vi "PH_Timing.panel.vi"(0 "object ref":refnum<vi>, 5 "error in (no error)":errorcluster) -> (19 "error out":errorcluster)   [LabVIEW 2014, in "PH_Timing.lvlib"]
doc: "This a GUI.\n\nLicense Agreement for this software:\n\nCopyright (C)\nGesellschaft für Schwerionenforschung, GSI\nPlanckstr. 1\n64291 Darmstadt\nGermany\n\nContact: D.Beck@gsi.de \n\nThis program is free software; you can redistribute it and/or modify it under the terms of the GNU General Public License as published by the Free Software Foundation; either version 2 of the license, or (at your option) any later version.\n\nThis program is distributed in the hope that it will be useful, but WITHOUT ANYW ARRANTY; without even the implied warranty of MERCHANTABILITY or FITNESS FOR A PARTICULAR PURPOSE. See the GNU General License for more details (http://www.gnu.org).\n\nGesellschaft für Schwerionenforschung, GSI\nPlanckstr. 1, 64291 Darmstadt, Germany\nFor all questions and ideas contact: M.Richter@gsi.de, H.Brand@gsi.de or D.Beck@gsi.de.\nLast update: 18-DEC-2002"
uses:
  PH_Timing.lvlib
  PH_StatusHandler/PH_StatusHandler.GUI element.ctl
  PH_Timing.PU Info.ctl
  PH_Timing.GateGen.ctl
  PH_Timing.Roughtuner.ctl
  PH_Timing.0.5HzGater.ctl
  PH_Timing.Slow Trigger Settings.ctl
  PH_Timing.Timing Mode.ctl
  PH_Timing.ns Generator.ctl
  instr.lib/Stanford Research DG645/Driver/Channel.ctl
  PH_SRDG645/PH_SRDG645.Channel Settings.ctl
  PH_Timing.Phase FEs.ctl
  CSCore/CSObj/CSObj.lvlib
  PH_Common/PH_Common.lvlib
  PH_Class/PH_Class.lvlib
  PH_StatusHandler/PH_StatusHandler.lvlib
  instr.lib/Stanford Research DG645/Stanford Research DG645 - Driver.lvlib
  PH_SRDG645/PH_SRDG645.lvlib
panel:
  out "FE Phase":T1 {"Phase" format="%#_12p"}
  out "Timing_ns_Ring_Regen_GD":u32(colorbox)=6618880 caption="ns Ring Regen"
  out "Timing Mode":T2 {"T2" min=0 max=6000 step=2}
  out "Slow Trigger Settings":T3
  out "Timing_0-5HzGater_GD":u32(colorbox)=6618880 caption="0.5Hz Gater"
  out "Timing_Roughtuner_GD":u32(colorbox)=6618880 caption="Roughtuner"
  out "Interlock Bypass":u32(colorbox)=6618880
  in  "Tab Control":T4(tab)
  out "ns Generator Settings":T5={"Instance"="N/A", "Phase fs / ns FE"={"Channel"=0, "Settings"={"Delay [s]"=0.0, "relative to"=0}}} {"Phase fs / ns FE"."Settings"."relative to" items=["T0", "T1", "A", "B", "C", "D", "E", "F", "G", "H"]; "Phase fs / ns FE"."Settings"."Delay [s]" format="%#_12p"; "Phase fs / ns FE"."Channel" items=["T0", "T1", "A", "B", "C", "D", "E", "F", "G", "H"]}
  out "Roughtuner Settings":T8={"Instance"="N/A", "Phase PHELIX / UNILAC"={"Channel"=0, "relative to"=0, "Delay [ms]"=0.0}, "Pulse Length"={"Channel"=0, "relative to"=0, "Delay [ms]"=0.0}, "Trigger"={"externally?"=FALSE, "Rate [Hz]"=0.0}} {"Pulse Length"."Delay [ms]" format="%#_8g"; "Pulse Length"."relative to" items=["T0", "A", "B", "AB", "C", "D", "CD"]; "Pulse Length"."Channel" items=["T0", "A", "B", "AB", "C", "D", "CD"]; "Phase PHELIX / UNILAC"."Delay [ms]" format="%#_8g"; "Phase PHELIX / UNILAC"."relative to" items=["T0", "A", "B", "AB", "C", "D", "CD"]; "Phase PHELIX / UNILAC"."Channel" items=["T0", "A", "B", "AB", "C", "D", "CD"]}
  out "Info 0,5Hz Gater":T9={"Instance"="N/A", "Channel ns FE Delay"=1, "Channel 0.5Hz"=1, "Width ns FE Delay"=1.0, "Width 0.5Hz"=1.0, "Delay ns FE Delay"=0.0, "Delay 0.5Hz"=0.0, "ns FE Delay active"=FALSE, "0.5Hz activ"=FALSE, "ns FE Delay inverted"=FALSE, "0.5Hz inverted"=FALSE} {"Channel ns FE Delay" items=["System (To)", "Channel A", "Channel B", "Channel C", "Channel D", "Channel E", "Channel F", "Channel G", "Channel H"]; "Channel 0.5Hz" items=["System (To)", "Channel A", "Channel B", "Channel C", "Channel D", "Channel E", "Channel F", "Channel G", "Channel H"]}
  out "Info Gate Generator":T10={"Instance"="N/A", "Channel Gate"=1, "Channel T2"=1, "Width Gate"=1.0, "Width T2"=1.0, "Delay Gate"=0.0, "Delay T2"=0.0, "Gate activ"=FALSE, "T2 activ"=FALSE, "System Mode"=enum."Normal"} {"Channel Gate" items=["System (To)", "Channel A", "Channel B", "Channel C", "Channel D", "Channel E", "Channel F", "Channel G", "Channel H"]; "Channel T2" items=["System (To)", "Channel A", "Channel B", "Channel C", "Channel D", "Channel E", "Channel F", "Channel G", "Channel H"]}
  out "PU PA 45-DP":T11={"Act CH?"=FALSE, "GD"="N/A", "CH"=1, "Delay"=99999.0, "active"=FALSE, "in Use?"=FALSE} {"CH" items=["System (To)", "Channel A", "Channel B", "Channel C", "Channel D", "Channel E", "Channel F", "Channel G", "Channel H"]; "Delay" format="%#_7f"}
  out "PU PA 45-MAIN":T11={"Act CH?"=FALSE, "GD"="N/A", "CH"=1, "Delay"=99999.0, "active"=FALSE, "in Use?"=FALSE} {"CH" items=["System (To)", "Channel A", "Channel B", "Channel C", "Channel D", "Channel E", "Channel F", "Channel G", "Channel H"]; "Delay" format="%#_7f"}
  out "PU PA 45-PILC":T11={"Act CH?"=FALSE, "GD"="N/A", "CH"=1, "Delay"=99999.0, "active"=FALSE, "in Use?"=FALSE} {"CH" items=["System (To)", "Channel A", "Channel B", "Channel C", "Channel D", "Channel E", "Channel F", "Channel G", "Channel H"]; "Delay" format="%#_7f"}
  out "PU PA 19-2":T11={"Act CH?"=FALSE, "GD"="N/A", "CH"=1, "Delay"=99999.0, "active"=FALSE, "in Use?"=FALSE} {"CH" items=["System (To)", "Channel A", "Channel B", "Channel C", "Channel D", "Channel E", "Channel F", "Channel G", "Channel H"]; "Delay" format="%#_7f"}
  out "PU PA 19-1":T11={"Act CH?"=FALSE, "GD"="N/A", "CH"=1, "Delay"=99999.0, "active"=FALSE, "in Use?"=FALSE} {"CH" items=["System (To)", "Channel A", "Channel B", "Channel C", "Channel D", "Channel E", "Channel F", "Channel G", "Channel H"]; "Delay" format="%#_7f"}
  out "PU MA 5":T11={"Act CH?"=FALSE, "GD"="N/A", "CH"=1, "Delay"=99999.0, "active"=FALSE, "in Use?"=FALSE} {"CH" items=["System (To)", "Channel A", "Channel B", "Channel C", "Channel D", "Channel E", "Channel F", "Channel G", "Channel H"]; "Delay" format="%#_7f"}
  out "PU MA 4":T11={"Act CH?"=FALSE, "GD"="N/A", "CH"=1, "Delay"=99999.0, "active"=FALSE, "in Use?"=FALSE} {"CH" items=["System (To)", "Channel A", "Channel B", "Channel C", "Channel D", "Channel E", "Channel F", "Channel G", "Channel H"]; "Delay" format="%#_7f"}
  out "PU MA 3":T11={"Act CH?"=FALSE, "GD"="N/A", "CH"=1, "Delay"=99999.0, "active"=FALSE, "in Use?"=FALSE} {"CH" items=["System (To)", "Channel A", "Channel B", "Channel C", "Channel D", "Channel E", "Channel F", "Channel G", "Channel H"]; "Delay" format="%#_7f"}
  out "PU MA 2":T11={"Act CH?"=FALSE, "GD"="N/A", "CH"=1, "Delay"=99999.0, "active"=FALSE, "in Use?"=FALSE} {"CH" items=["System (To)", "Channel A", "Channel B", "Channel C", "Channel D", "Channel E", "Channel F", "Channel G", "Channel H"]; "Delay" format="%#_7f"}
  out "PU MA 1":T11={"Act CH?"=FALSE, "GD"="N/A", "CH"=1, "Delay"=99999.0, "active"=FALSE, "in Use?"=FALSE} {"CH" items=["System (To)", "Channel A", "Channel B", "Channel C", "Channel D", "Channel E", "Channel F", "Channel G", "Channel H"]; "Delay" format="%#_7f"}
  out "PA MA FR":T11={"Act CH?"=FALSE, "GD"="N/A", "CH"=1, "Delay"=99999.0, "active"=FALSE, "in Use?"=FALSE} {"CH" items=["System (To)", "Channel A", "Channel B", "Channel C", "Channel D", "Channel E", "Channel F", "Channel G", "Channel H"]; "Delay" format="%#_7f"}
  out "State Sequencer":string caption="State PU"
  out "Timing_PP_2_GD":u32(colorbox)=6618880 caption="PP 2"
  out "Timing_PP_1_GD":u32(colorbox)=6618880 caption="PP 1"
  out "Status":T12 caption="Enabling State"
  in  "Delete":bool
  out "Timing_GateGen_GD":u32(colorbox)=6618880 caption="GateGen"
  in  "Exit":bool
  # "PCS"
  # "3.40"
  # "AND ns FE Delay"
  # "AND 0.5 Hz"
  # "Gate"
  # "T2"
  # "s"
  # "s"
  # "s"
  # "s"
  # "s"
  # "s"
  # "s"
  # "s"
  # "s"
  # "s"
  # "s"
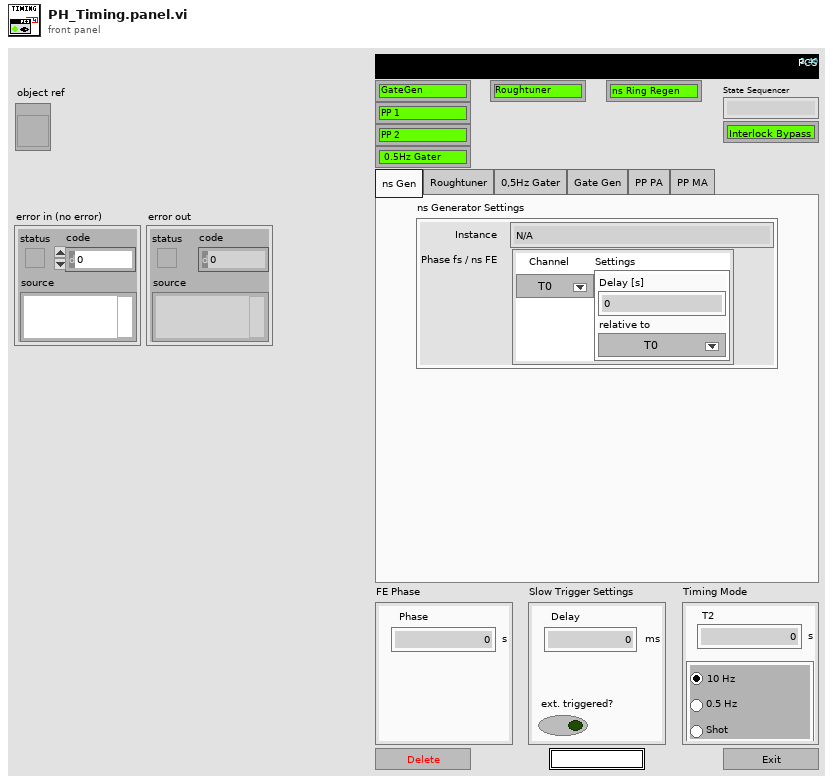
[diagram p1: front panel]
types:
  T1 = typedef "PH_Timing.lvlib/PH_Timing.Phase FEs.ctl" = cluster{"Phase":dbl}
  T2 = typedef "PH_Timing.lvlib/PH_Timing.Timing Mode.ctl" = cluster{"T2":i16, "Modeselector":enum32{"10 Hz", "0.5 Hz", "Shot"}}
  T3 = typedef "PH_Timing.lvlib/PH_Timing.Slow Trigger Settings.ctl" = cluster{"Delay":dbl, "externally triggered?":bool}
  T4 = enum32{"ns Gen", "Roughtuner", "0,5Hz Gater", "Gate Gen", "PP PA", "PP MA"}
  T5 = typedef "PH_Timing.lvlib/PH_Timing.ns Generator.ctl" = cluster{"Instance":string, "Phase fs / ns FE":cluster{"Channel":T6, "Settings":T7}}
  T6 = typedef "Stanford Research DG645 - Driver.lvlib/Channel.ctl" = i32
  T7 = typedef "PH_SRDG645.lvlib/PH_SRDG645.Channel Settings.ctl" = cluster{"Delay [s]":dbl, "relative to":i32}
  T8 = typedef "PH_Timing.lvlib/PH_Timing.Roughtuner.ctl" = cluster{"Instance":string, "Phase PHELIX / UNILAC":cluster{"Channel":u16, "relative to":u16, "Delay [ms]":dbl}, "Pulse Length":cluster{"Channel":u16, "relative to":u16, "Delay [ms]":dbl}, "Trigger":cluster{"externally?":bool, "Rate [Hz]":dbl}}
  T9 = typedef "PH_Timing.lvlib/PH_Timing.0.5HzGater.ctl" = cluster{"Instance":string, "Channel ns FE Delay":i32, "Channel 0.5Hz":i32, "Width ns FE Delay":dbl, "Width 0.5Hz":dbl, "Delay ns FE Delay":dbl, "Delay 0.5Hz":dbl, "ns FE Delay active":bool, "0.5Hz activ":bool, "ns FE Delay inverted":bool, "0.5Hz inverted":bool}
  T10 = typedef "PH_Timing.lvlib/PH_Timing.GateGen.ctl" = cluster{"Instance":string, "Channel Gate":i32, "Channel T2":i32, "Width Gate":dbl, "Width T2":dbl, "Delay Gate":dbl, "Delay T2":dbl, "Gate activ":bool, "T2 activ":bool, "System Mode":enum16{"Normal", "Single", "Burst", "Duty Cycle"}}
  T11 = typedef "PH_Timing.lvlib/PH_Timing.PU Info.ctl" = cluster{"Act CH?":bool, "GD":string, "CH":i32, "Delay":dbl, "active":bool, "in Use?":bool}
  T12 = typedef "PH_StatusHandler.lvlib/PH_StatusHandler.GUI element.ctl" = u16
  T13 = cluster{"MA PU 1":refnum<vi>, "MA PU 2":refnum<vi>, "MA PU 3":refnum<vi>, "MA PU 4":refnum<vi>, "MA PU 5":refnum<vi>, "MA FR":refnum<vi>, "PA 19mm 1":refnum<vi>, "PA 19mm 2":refnum<vi>, "PA 45mm PILC":refnum<vi>, "PA 45mm MAIN":refnum<vi>, "PA 45mm DP":refnum<vi>}
  T14 = typedef "PH_Timing.lvlib/PH_Timing.PU Data.ctl" = cluster{"linked?":bool, "Data":T11, "GD":cluster{"Device Status":T15, "linked?":bool}, "GUI Ref":refnum<vi>, "PU":T16}
  T15 = typedef "PH_StatusHandler.lvlib/PH_StatusHandler.Status.ctl" = i16
  T16 = typedef "PH_PP_Common.lvlib/PH_PP_Common.PUs.ctl" = enum16{"no Info", "PA-19mm-1", "PA-19mm-2", "PA-45mm-PILC", "PA-45mm-MAIN", "MA-PU-1", "MA-PU-2", "MA-PU-3", "MA-PU-4", "MA-PU-5", "MA-PU-6", "MA-FR", "MA-PILC", "PA-45mm-DP"}
  T17 = typedef "PH_Timing.lvlib/PH_Timing.i attribute.ctl" = cluster{"Sequencer":cluster{"linked?":bool, "Proc State":string, "Ref State":refnum<vi>}, "Gate Generator":cluster{"GD":cluster{"Device Status":T15, "linked?":bool}, "Settings":T10, "GUI Ref":refnum<vi>}, "Interlock Bypass":cluster{"Instancename":string, "Switch linked?":bool, "Device Status":T15, "Ref Status":refnum<vi>}, "Roughtuner":cluster{"Settings":T8, "GUI Ref":refnum<vi>, "GD":cluster{"Device Status":T15, "linked?":bool}}, "0,5Hz Gater":cluster{"Settings":T9, "GUI Ref":refnum<vi>, "GD":cluster{"Device Status":T15, "linked?":bool}}, "Slow Trigger":cluster{"Settings":T3, "GUI Ref":refnum<vi>, "Service ID Delay":i32, "Service ID Ext Trig":i32, "Wanted Settings":T3}, "Timing Mode":cluster{"Mode":T2, "GUI Ref":refnum<vi>, "Service ID T2":i32, "Service ID Mode":i32, "Wanted Mode":T2}, "ns Generator":cluster{"Settings":T5, "ns Generator Settings":refnum<vi>, "GD":cluster{"Device Status":T15, "linked?":bool}}, "Phase FEs":cluster{"Settings":T1, "GUI Ref":refnum<vi>, "Service ID Phase":i32, "Wanted Settings":T1}, "GD GUI Refs":refnum<vi>[], "Heads":T14[], "GUI Ref Delete":refnum<vi>}
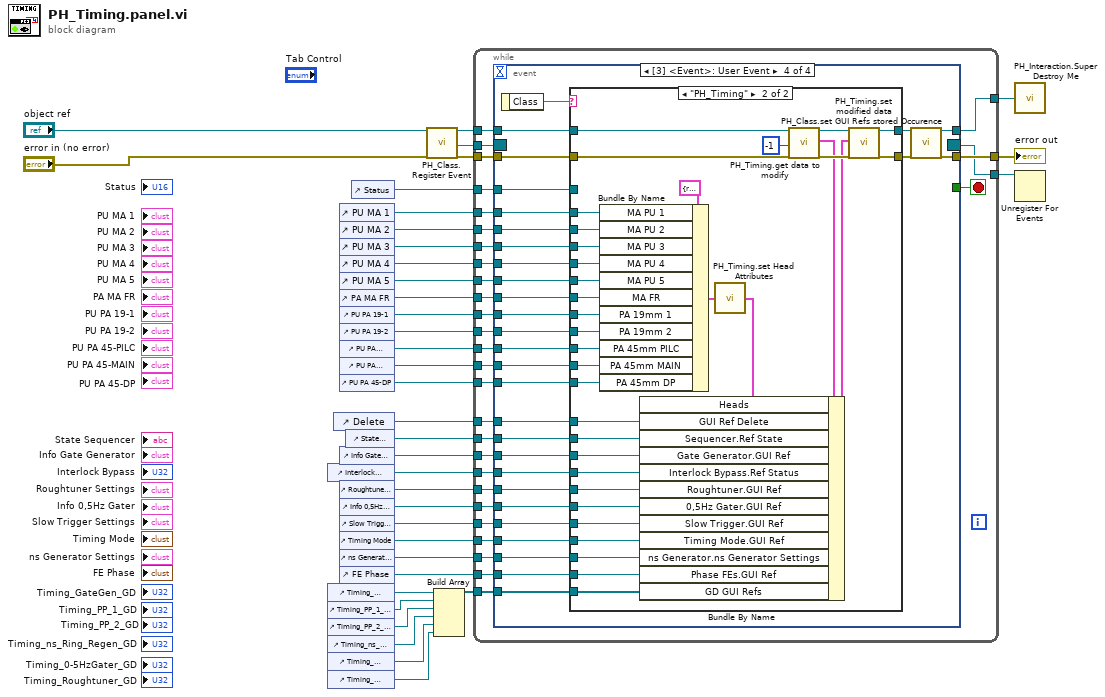
[diagram p0: block diagram]
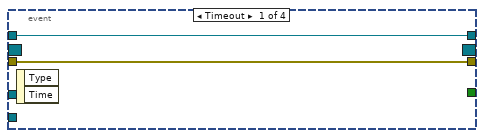
[diagram p2: hidden frame]
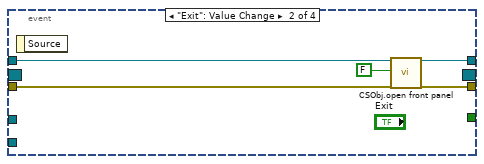
[diagram p3: hidden frame]
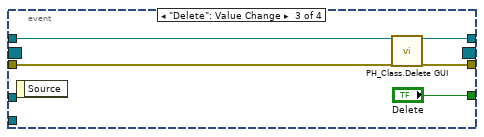
[diagram p4: hidden frame]
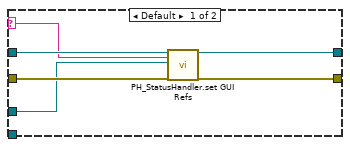
[diagram p5: hidden frame]
diagram:
  n1 = control-ref of="Interlock Bypass"() -> (w9:refnum<vi>)
  n2 = control-ref of="Timing_GateGen_GD"() -> (w37:refnum<vi>)
  n3 = control-ref of="Timing_PP_1_GD"() -> (w36:refnum<vi>)
  n4 = control-ref of="Timing_PP_2_GD"() -> (w35:refnum<vi>)
  n5 = control-ref of="Timing_ns_Ring_Regen_GD"() -> (w31:refnum<vi>)
  n6 = control-ref of="Timing_0-5HzGater_GD"() -> (w32:refnum<vi>)
  n7 = control-ref of="Timing_Roughtuner_GD"() -> (w30:refnum<vi>)
  n8 = control-ref of="Delete"() -> (w12:refnum<vi>)
  n9 = control-ref of="PU MA 1"() -> (w23:refnum<vi>)
  n10 = control-ref of="PU MA 2"() -> (w22:refnum<vi>)
  n11 = control-ref of="PU MA 3"() -> (w21:refnum<vi>)
  n12 = control-ref of="PU MA 4"() -> (w20:refnum<vi>)
  n13 = control-ref of="PU MA 5"() -> (w19:refnum<vi>)
  n14 = control-ref of="PA MA FR"() -> (w18:refnum<vi>)
  n15 = control-ref of="PU PA 19-1"() -> (w17:refnum<vi>)
  n16 = control-ref of="PU PA 19-2"() -> (w16:refnum<vi>)
  n17 = control-ref of="PU PA 45-PILC"() -> (w15:refnum<vi>)
  n18 = control-ref of="PU PA 45-MAIN"() -> (w14:refnum<vi>)
  n19 = control-ref of="PU PA 45-DP"() -> (w13:refnum<vi>)
  n20 = control-ref of="Info Gate Generator"() -> (w10:refnum<vi>)
  n21 = control-ref of="Roughtuner Settings"() -> (w8:refnum<vi>)
  n22 = control-ref of="Info 0,5Hz Gater"() -> (w7:refnum<vi>)
  n23 = control-ref of="Slow Trigger Settings"() -> (w6:refnum<vi>)
  n24 = control-ref of="Timing Mode"() -> (w5:refnum<vi>)
  n25 = control-ref of="ns Generator Settings"() -> (w4:refnum<vi>)
  n26 = control-ref of="FE Phase"() -> (w3:refnum<vi>)
  n27 = control-ref of="State Sequencer"() -> (w11:refnum<vi>)
  n28 = control-ref of="Status"() -> (w1:refnum<vi>)
  n29 = call "PH_Class.Register Event.vi"("i ref in"="object ref", "error in (no error)"="error in (no error)") -> ("i ref out"=w29:refnum<vi>, "Event Registration Refnum"=w27:refnum<event-registration>, "error out"=w28:errorcluster)  [unwired: 15 in]
  n30 = Build Array(w37, w36, w35, w31, w32, w30) -> (w2:refnum<vi>[])
  n31 = while {
    tunnel: w29 -> [w64]
    tunnel: [w63] -> w34
    tunnel: w28 -> [w66]
    tunnel: [w65] -> w33
    tunnel: w27 -> [w62]
    tunnel: [w61] -> w26
    tunnel: w23 -> [w60]
    tunnel: w22 -> [w59]
    tunnel: w21 -> [w58]
    tunnel: w20 -> [w57]
    tunnel: w19 -> [w56]
    tunnel: w18 -> [w55]
    tunnel: w17 -> [w54]
    tunnel: w16 -> [w53]
    tunnel: w15 -> [w52]
    tunnel: w14 -> [w51]
    tunnel: w13 -> [w50]
    tunnel: w12 -> [w49]
    tunnel: w1 -> [w48]
    tunnel: w11 -> [w47]
    tunnel: w10 -> [w46]
    tunnel: w9 -> [w45]
    tunnel: w8 -> [w44]
    tunnel: w7 -> [w43]
    tunnel: w6 -> [w42]
    tunnel: w5 -> [w41]
    tunnel: w4 -> [w40]
    tunnel: w3 -> [w39]
    tunnel: w2 -> [w38]
    stop <- w67 stop-if-true
    n32 = event shown="[3] <Event>: User Event" {
      selector: w62 -> [_ _ _ _]
      dyn-events: [_ _ _ _] -> w61
      timeout: _ -> [_ _ _ _]
      tunnel: [_ _ "Delete" _] -> w67
      tunnel: w64 -> [w68 w74 w76 w107]
      tunnel: w66 -> [w69 w72 w78 w105]
      tunnel: [w69 w71 w77 w108] -> w65
      tunnel: [w68 w70 w75 w109] -> w63
      tunnel: w60 -> [_ _ _ w102]
      tunnel: w59 -> [_ _ _ w101]
      tunnel: w58 -> [_ _ _ w100]
      tunnel: w57 -> [_ _ _ w99]
      tunnel: w56 -> [_ _ _ w98]
      tunnel: w55 -> [_ _ _ w97]
      tunnel: w54 -> [_ _ _ w96]
      tunnel: w53 -> [_ _ _ w95]
      tunnel: w52 -> [_ _ _ w94]
      tunnel: w51 -> [_ _ _ w93]
      tunnel: w50 -> [_ _ _ w92]
      tunnel: w49 -> [_ _ _ w91]
      tunnel: w48 -> [_ _ _ w90]
      tunnel: w47 -> [_ _ _ w89]
      tunnel: w46 -> [_ _ _ w88]
      tunnel: w45 -> [_ _ _ w87]
      tunnel: w44 -> [_ _ _ w86]
      tunnel: w43 -> [_ _ _ w85]
      tunnel: w42 -> [_ _ _ w84]
      tunnel: w41 -> [_ _ _ w83]
      tunnel: w40 -> [_ _ _ w82]
      tunnel: w39 -> [_ _ _ w81]
      tunnel: w38 -> [_ _ _ w80]
      event Timeout {
        n33 = event-data() -> ()  [unwired: 1 in, 2 out]
      }
      event "Exit": Value Change {
        n34 = event-data() -> ()  [unwired: 1 in, 1 out]
        n35 = call "CSObj.open front panel.vi"("i ref in"=w74, "frontPanelOpen"=FALSE ("front panel open"), "error in (no error)"=w72) -> ("i ref out"=w70:refnum<vi>, "error out"=w71:errorcluster)  [unwired: 15 in]
      }
      event "Delete": Value Change {
        n36 = event-data() -> ()  [unwired: 1 in, 1 out]
        n37 = call "PH_Class.Delete GUI.vi"("VI in"=w76, "error in (no error)"=w78) -> ("VI out"=w75:refnum<vi>, "error out"=w77:errorcluster)  [unwired: 16 in]
      }
      event User Event {
        n38 = event-data() -> ("Class"=w103:string)  [unwired: 1 in]
        n39 = case shown="\"PH_Timing\"" w103 {
          selector: w103 -> [w111 _]
          tunnel: w107 -> [w113 w116]
          tunnel: [w112 w141] -> w106
          tunnel: w105 -> [w115 w117]
          tunnel: [w114 w140] -> w104
          tunnel: w102 -> [_ w139]
          tunnel: w101 -> [_ w138]
          tunnel: w100 -> [_ w137]
          tunnel: w99 -> [_ w136]
          tunnel: w98 -> [_ w135]
          tunnel: w97 -> [_ w134]
          tunnel: w96 -> [_ w133]
          tunnel: w95 -> [_ w132]
          tunnel: w94 -> [_ w131]
          tunnel: w93 -> [_ w130]
          tunnel: w92 -> [_ w129]
          tunnel: w91 -> [_ w128]
          tunnel: w90 -> [w110 _]
          tunnel: w89 -> [_ w127]
          tunnel: w88 -> [_ w126]
          tunnel: w87 -> [_ w125]
          tunnel: w86 -> [_ w124]
          tunnel: w85 -> [_ w123]
          tunnel: w84 -> [_ w122]
          tunnel: w83 -> [_ w121]
          tunnel: w82 -> [_ w120]
          tunnel: w81 -> [_ w119]
          tunnel: w80 -> [_ w118]
          frame Default {
            n40 = call "PH_StatusHandler.set GUI Refs.vi"("i ref in"=w113, "Class"=w111, "GUI Ref"=w110, "error in (no error)"=w115) -> ("i ref out"=w112:refnum<vi>, "error out"=w114:errorcluster)  [unwired: 14 in]
          }
          frame "PH_Timing" {
            n41 = Bundle By Name(cluster=T13 {"MA PU 1"=refnum, "MA PU 2"=refnum, "MA PU 3"=refnum, "MA PU 4"=refnum, "MA PU 5"=refnum, "MA FR"=refnum, "PA 19mm 1"=refnum, "PA 19mm 2"=refnum, "PA 45mm PILC"=refnum, "PA 45mm MAIN"=refnum, "PA 45mm DP"=refnum} ("GUI Refs Heads"), "MA PU 1"=w139, "MA PU 2"=w138, "MA PU 3"=w137, "MA PU 4"=w136, "MA PU 5"=w135, "MA FR"=w134, "PA 19mm 1"=w133, "PA 19mm 2"=w132, "PA 45mm PILC"=w131, "PA 45mm MAIN"=w130, "PA 45mm DP"=w129) -> (w142:T13)
            n42 = call "PH_Timing.set Head Attributes.vi"("GUI Refs Heads"=w142) -> ("Heads"=w144:T14[])
            n43 = call "PH_Timing.get data to modify.vi"("i ref in"=w116, "ms timeout (10000)"=-1, "error in (no error)"=w117) -> ("i ref out"=w149:refnum<vi>, "i attribute"=w145:T17, "error out"=w148:errorcluster)  [unwired: 13 in, 1 out]
            n44 = Bundle By Name(cluster=w145, "Heads"=w144, "GUI Ref Delete"=w128, "Sequencer.Ref State"=w127, "Gate Generator.GUI Ref"=w126, "Interlock Bypass.Ref Status"=w125, "Roughtuner.GUI Ref"=w124, "0,5Hz Gater.GUI Ref"=w123, "Slow Trigger.GUI Ref"=w122, "Timing Mode.GUI Ref"=w121, "ns Generator.ns Generator Settings"=w120, "Phase FEs.GUI Ref"=w119, "GD GUI Refs"=w118) -> (w147:T17)
            n45 = call "PH_Timing.set modified data.vi"("i ref in"=w149, "i attribute"=w147, "error in (no error)"=w148) -> ("i ref out"=w141:refnum<vi>, "error out"=w140:errorcluster)  [unwired: 15 in]
          }
        }
        n46 = call "PH_Class.set GUI Refs stored Occurence.vi"("i ref in"=w106, "error in (no error)"=w104) -> ("i ref out"=w109:refnum<vi>, "error out"=w108:errorcluster)  [unwired: 16 in]
      }
    }
  }
  "error out" <- w33
  n47 = call "PH_Interaction.Super Destroy Me.vi"("i ref out"=w34) -> ()
  n48 = Unregister For Events(event registration refnum=w26) -> ()  [unwired: 1 in, 1 out]
